vi "Measure.vi"() -> ()   [LabVIEW 2015]
uses:
  <vilib>/Utility/error.llb/DialogType.ctl
  <vilib>/DAQmx/write.llb/DAQmx Write (Analog 1D Wfm NChan NSamp).vi
  <vilib>/DAQmx/read.llb/DAQmx Read (Analog 1D Wfm NChan NSamp).vi
  <vilib>/DAQmx/create/channels.llb/DAQmx Create Channel (AO-Voltage-Basic).vi
  <vilib>/DAQmx/configure/timing.llb/DAQmx Timing (Sample Clock).vi
  <vilib>/DAQmx/create/channels.llb/DAQmx Create Channel (AI-Voltage-Basic).vi
  <vilib>/DAQmx/configure/trigger.llb/DAQmx Start Trigger (Digital Edge).vi
  <vilib>/DAQmx/miscellaneous.llb/DAQmx Fill In Error Info.vi
  <vilib>/measure/NI_MABase.lvlib
  <resource>/objmgr/daqmx.rc
panel:
  out "Waveform Chart":waveform(dbl)[](graph)
  in  "Samples to Read":i32=1000
  in  "rate":dbl=5000.0 caption="Update Generation Rate" format="%0.2f"
  in  "minimum value":dbl=-10.0 caption="Output Minimum Value" format="%0.2f"
  in  "maximum value":dbl=10.0 caption="Output Maximum Value" format="%0.2f"
  in  "Maximum Value":dbl=10.0 caption="Input Maximum Value" format="%0.2f"
  in  "Minimum Value":dbl=-10.0 caption="Input Minimum Value" format="%0.2f"
  in  "Rate":dbl=10000.0 caption="Input Rate" format="%0.2f"
  in  "?":bool
  in  "Fil lagres til":path
  in  "Ventetid(s)":u32
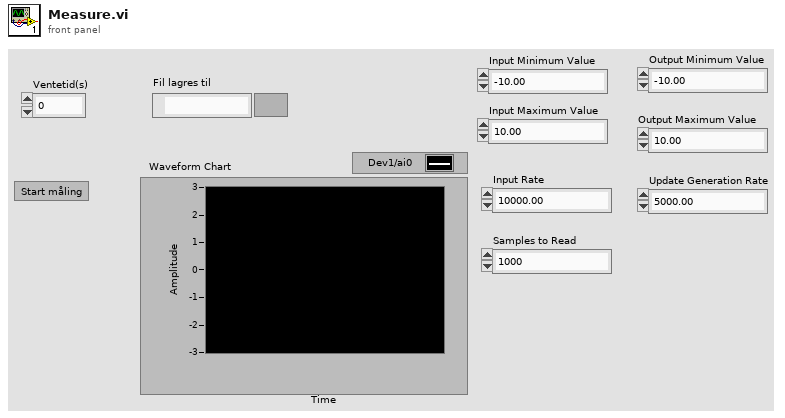
[diagram p1: front panel]
types:
  T1 = typedef "DialogType.ctl" = u16
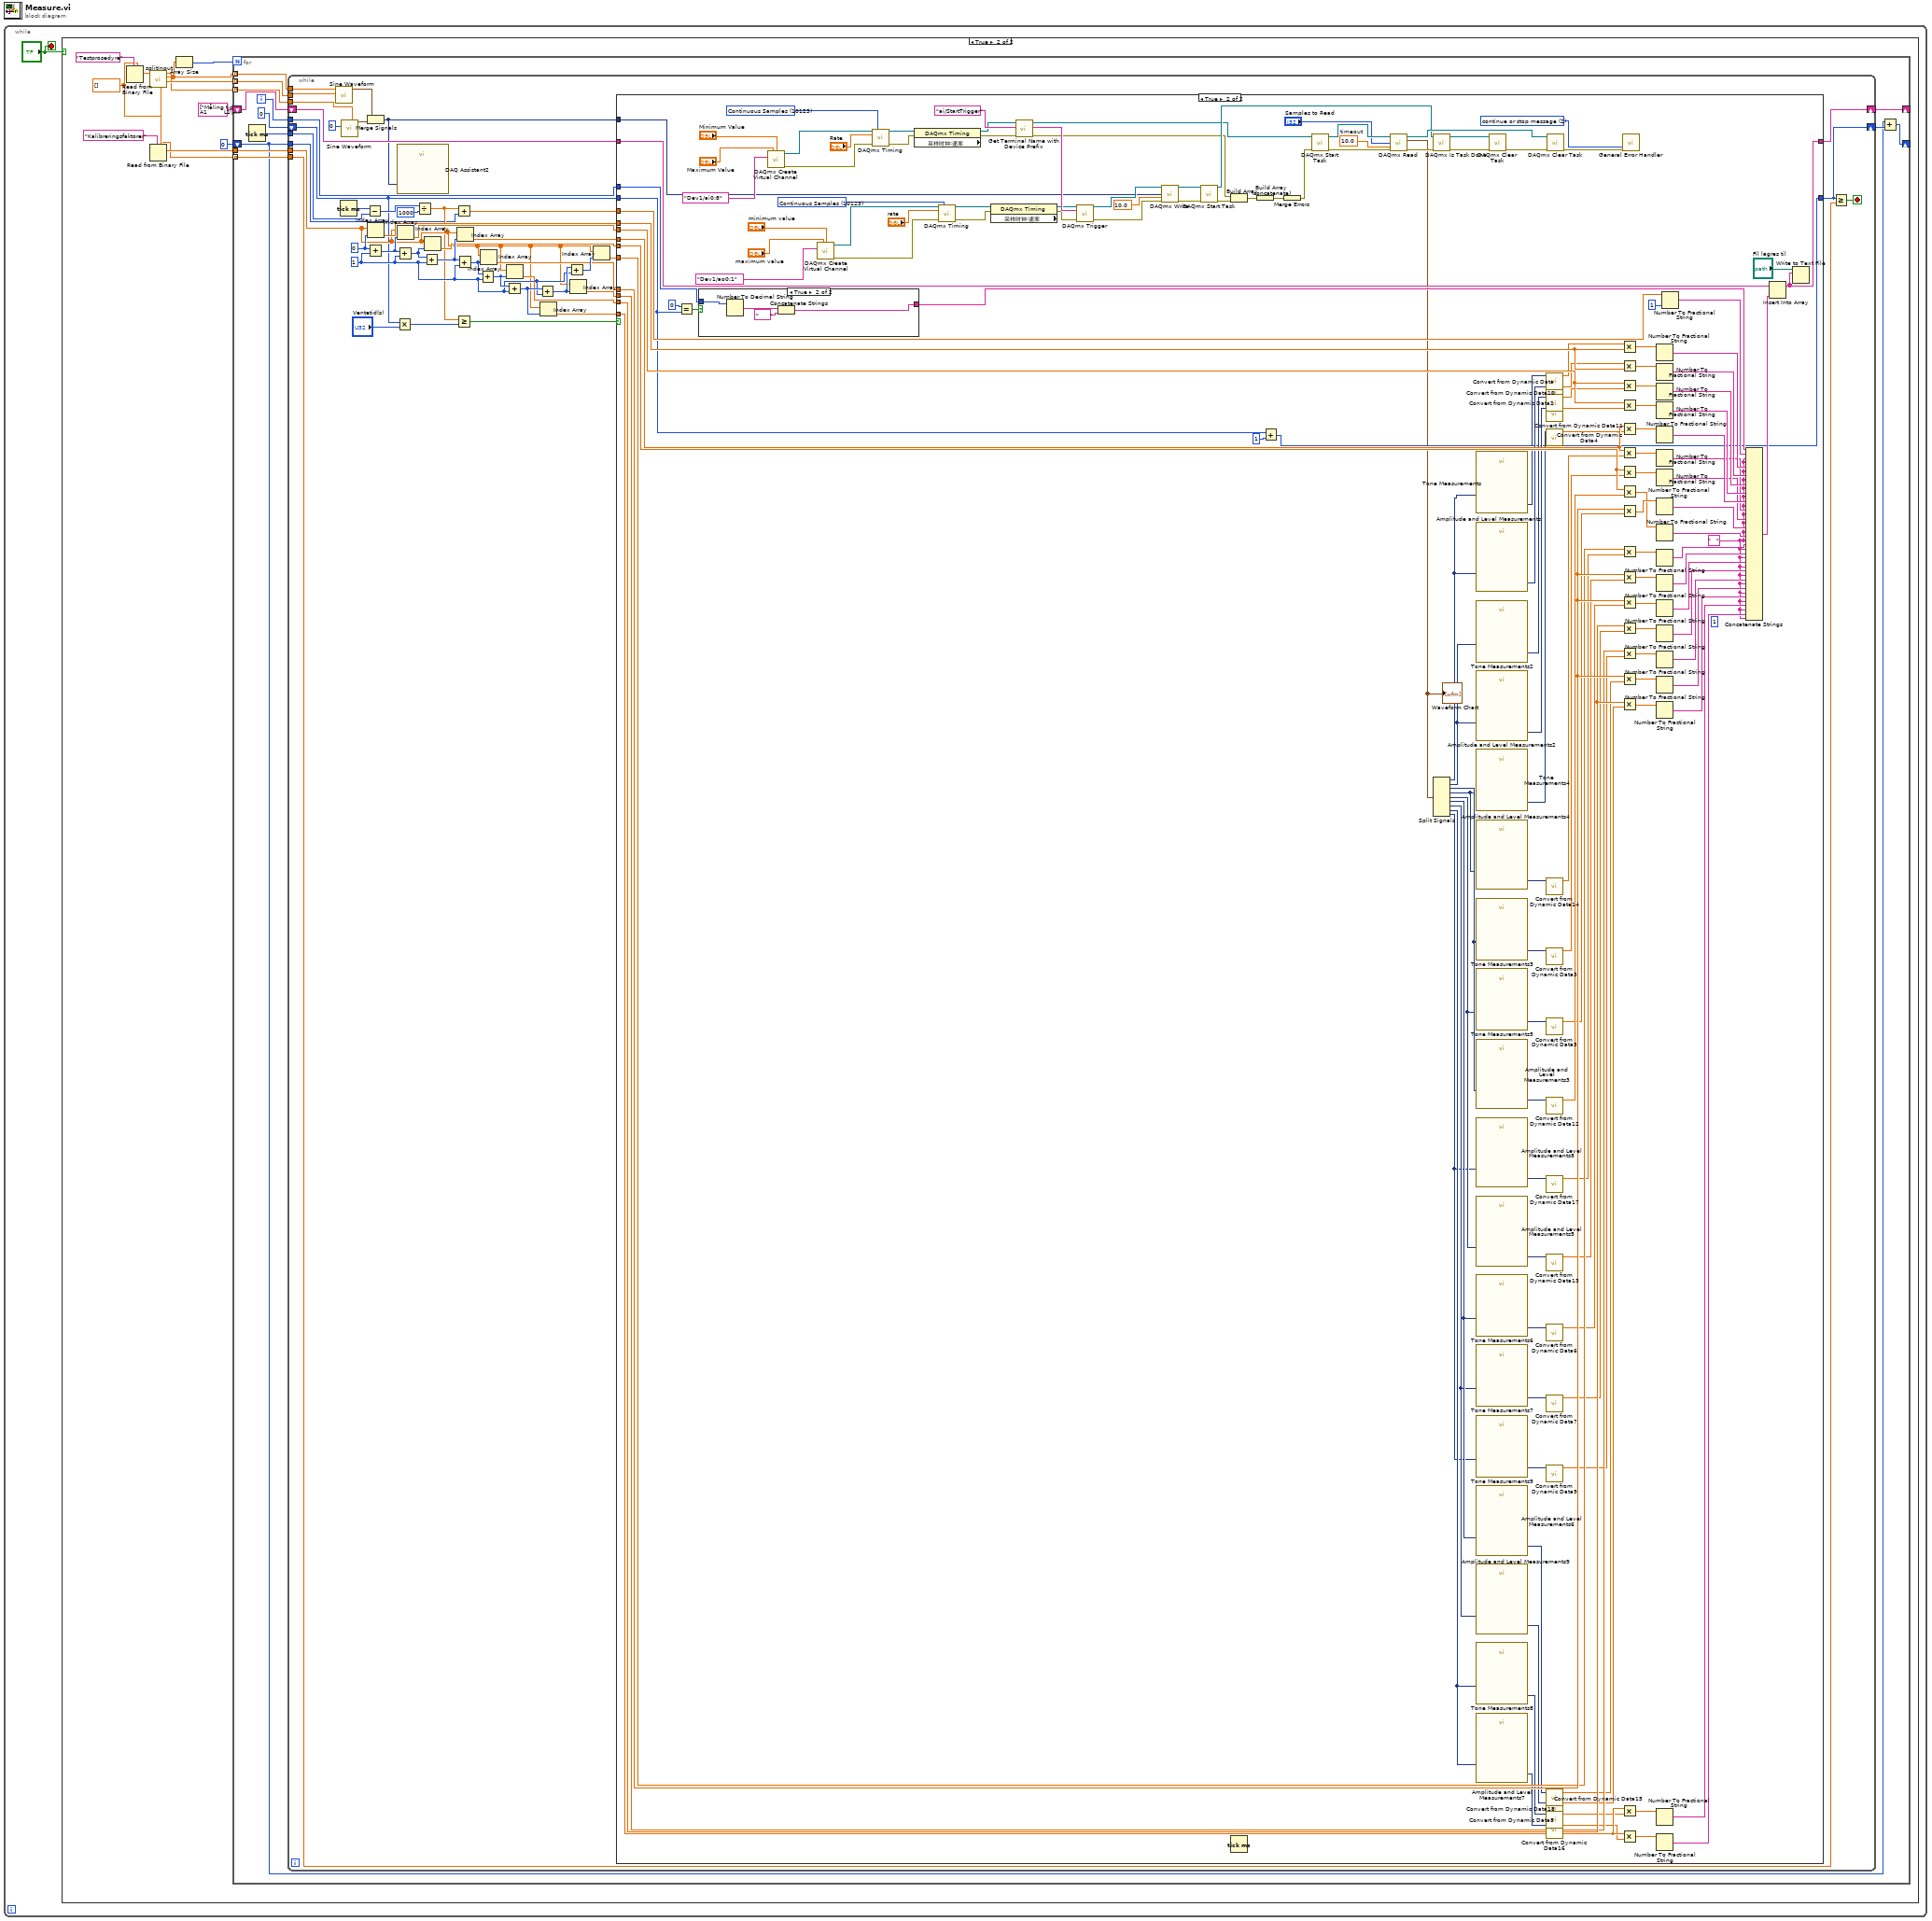
[diagram p0: block diagram]
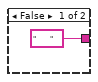
[diagram p4: hidden frame]
diagram:
  n1 = while {
    stop <- "?" stop-if-true
    n2 = case shown="True" "?" {
      frame False {
      }
      frame True {
        w9 = dbl[] [] ("Array")
        n3 = Read from Binary File(5:w9, 7:"Testprosedyre" ("String")) -> (2:w13:dbl[])  [unwired: 4 in, 3 out]
        n4 = call "splitInput.vi"("Array in"=w13) -> ("Amplitude"=w6:dbl[], "Frekvens"=w4:dbl[], "Temperatur"=w5:dbl[], "Perioder"=w7:dbl[])  [unwired: 7 in]
        n5 = Read from Binary File(5:w9, 7:"Kalibreringsfaktorer") -> (2:w8:dbl[])  [unwired: 4 in, 3 out]
        n6 = Array Size(array=w4) -> (size(s)=w11:i32)
        n7 = for {
          N: w11 -> [_]
          tunnel: w8 -> [w24]
          tunnel: w7 -> [w23] mode=indexing
          tunnel: w6 -> [w22] mode=indexing
          tunnel: w4 -> [w21] mode=indexing
          tunnel: w5 -> [w20] mode=indexing
          shift-right: [w18] -> _
          shift-left: string[] ["Måling tid       A1         L1\t       A2         L2         A3         L3         A4         L4         A5         L5         A6         L6         A7         L7         A8         L8         A9         L9"] ("Array") -> [w19]
          shift-right: [w14] -> _
          shift-left: 0 -> [w15]
          i -> [w25]
          n8 = Tick Count (ms)() -> (millisecond timer value=w17:u32)
          n9 = while {
            shift-right: [w42] -> w16
            shift-left: 0 -> [w36]
            shift-right: [w46] -> w18
            shift-left: w19 -> [w47]
            tunnel: w25 -> [w45]
            tunnel: w23 -> [w43]
            tunnel: w24 -> [w41]
            tunnel: w17 -> [w40]
            tunnel: w22 -> [w29]
            tunnel: w21 -> [w30]
            tunnel: w20 -> [w39]
            tunnel: w15 -> [w33]
            stop <- w44 stop-if-true
            w53 = 1
            w70 = 0
            n10 = call <vilib>:"Sine Waveform.vi"("amplitude"=w29, "frequency"=w30) -> ("signal out"=w27:waveform(dbl))  [unwired: 8 in, 1 out]
            n11 = Tick Count (ms)() -> (millisecond timer value=w50:u32)
            n12 = call <vilib>:"Sine Waveform.vi"("offset"=w39, "amplitude"=0) -> ("signal out"=w31:waveform(dbl))  [unwired: 8 in, 1 out]
            n13 = Subtract(x=w50, y=w40) -> (x-y=w49:u32)
            n14 = Add(x=w70, y=w53) -> (x+y=w52:i32)
            n15 = Merge Signals(w27, w31) -> (w32:dynamicdata)
            n16 = Index Array(array=w41, index=w70) -> (element=w62:dbl)
            n17 = Multiply(x=w36, y="Ventetid(s)") -> (x*y=w38:u32)
            n18 = Add(x=w52, y=w53) -> (x+y=w69:i32)
            n19 = call "DAQ Assistant2"("data"=w32) -> ()  [unwired: 17 in, 2 out]
            n20 = Index Array(array=w41, index=w52) -> (element=w61:dbl)
            n21 = Divide(x=w49, y=1000) -> (x/y=w34:dbl)
            n22 = Add(x=w69, y=w53) -> (x+y=w68:i32)
            n23 = Index Array(array=w41, index=w69) -> (element=w60:dbl)
            n24 = Add(x=w34, y=w33) -> (x+y=w35:dbl)
            n25 = Greater Or Equal?(x=w34, y=w38) -> (x >= y?=w48:bool)
            n26 = Add(x=w68, y=w53) -> (x+y=w67:i32)
            n27 = Index Array(array=w41, index=w68) -> (element=w59:dbl)
            n28 = Add(x=w67, y=w53) -> (x+y=w66:i32)
            n29 = Index Array(array=w41, index=w67) -> (element=w58:dbl)
            n30 = Add(x=w66, y=w53) -> (x+y=w65:i32)
            n31 = Index Array(array=w41, index=w66) -> (element=w57:dbl)
            n32 = Add(x=w65, y=w53) -> (x+y=w64:i32)
            n33 = Index Array(array=w41, index=w65) -> (element=w56:dbl)
            n34 = Add(x=w64, y=w53) -> (x+y=w63:i32)
            n35 = Index Array(array=w41, index=w64) -> (element=w55:dbl)
            n36 = Index Array(array=w41, index=w63) -> (element=w54:dbl)
            n37 = case shown="True" w48 {
              tunnel: w47 -> [w72 w226]
              tunnel: w62 -> [_ w225]
              tunnel: w61 -> [_ w224]
              tunnel: w60 -> [_ w223]
              tunnel: w59 -> [_ w222]
              tunnel: w58 -> [_ w221]
              tunnel: w57 -> [_ w220]
              tunnel: w56 -> [_ w219]
              tunnel: w55 -> [_ w218]
              tunnel: w54 -> [_ w217]
              tunnel: w35 -> [_ w129]
              tunnel: w36 -> [w71 w125]
              tunnel: [w72 w128] -> w46
              tunnel: w45 -> [_ w126]
              tunnel: [w71 w124] -> w42
              tunnel: w32 -> [_ w76]
              frame False {
              }
              frame True {
                (unwired) 1
                w79 = 10.0  # timeout
                w102 = T1 2 items=["no dialog", "OK message", "continue or stop message", "OK message + warnings", "continue/stop + warnings"] ("type of dialog (OK msg:1)")
                w114 = 10123 items=["Finite Samples"=10178, "Continuous Samples"=10123] ("sample mode")
                w120 = 10123 items=["Finite Samples"=10178, "Continuous Samples"=10123] ("sample mode")
                w130 = "   "
                n38 = Equal?(x=0, y=w125) -> (x = y?=w171:bool)
                n39 = case shown="True" w171 {
                  tunnel: ["       " w229] -> w151
                  tunnel: w126 -> [_ w228]
                  frame False {
                  }
                  frame True {
                    n40 = Number To Decimal String(number=w228) -> (decimal integer string=w231:string)  [unwired: 1 in]
                    n41 = Concatenate Strings(w231, "      ") -> (w229:string)
                  }
                }
                n42 = call-poly <vilib>:"DAQmx Create Virtual Channel.vi"("maximum value"="Maximum Value", "minimum value"="Minimum Value", "physical channels"=tag "Dev1/ai0:8" ("Physical Channel")) -> ("task out"=w118:refnum<k21>, "error out"=w119:errorcluster)  [unwired: 11 in]
                n43 = call-poly <vilib>:"DAQmx Create Virtual Channel.vi"("maximum value"="maximum value", "minimum value"="minimum value", "physical channels"=tag "Dev1/ao0:1") -> ("task out"=w113:refnum<k21>, "error out"=w112:errorcluster)  [unwired: 11 in]
                n44 = call-poly <vilib>:"DAQmx Timing.vi"("task/channels in"=w118, "sample mode"=w120, "rate"="Rate", "error in"=w119) -> ("task out"=w88:refnum<k21>, "error out"=w87:errorcluster)  [unwired: 10 in]
                n45 = property class="DAQmx Timing" props=["采样时钟:速率"](reference=w88, error in=w87) -> (reference out=w86:refnum<k21>, error out=w85:errorcluster)  [unwired: 1 out]
                n46 = call-poly <vilib>:"DAQmx Timing.vi"("task/channels in"=w113, "sample mode"=w114, "rate"="rate", "error in"=w112) -> ("task out"=w97:refnum<k21>, "error out"=w96:errorcluster)  [unwired: 10 in]
                n47 = property class="DAQmx Timing" props=["采样时钟:速率"](reference=w97, error in=w96) -> (reference out=w98:refnum<k21>, error out=w95:errorcluster)  [unwired: 1 out]
                n48 = call "Get Terminal Name with Device Prefix.vi"("error in (no error)"=w85, "Local Terminal Name"="ai/StartTrigger" ("terminal"), "task/channels in"=w86) -> ("error out"=w92:errorcluster, "Terminal Name with Device Prefix"=w99:tag, "task out"=w94:refnum<k21>)  [unwired: 6 in]
                n49 = call-poly <vilib>:"DAQmx Trigger.vi"("task/channels in"=w98, "source"=w99, "error in"=w95) -> ("task out"=w104:refnum<k21>, "error out"=w105:errorcluster)  [unwired: 11 in]
                n50 = call-poly <vilib>:"DAQmx Write.vi"("task/channels in"=w104, "data"=w76, "timeout"=10.0 ("Wirite Timeout"), "error in"=w105) -> ("task out"=w107:refnum<k21>, "error out"=w106:errorcluster)  [unwired: 9 in, 1 out]
                n51 = call <vilib>:"DAQmx Start Task.vi"("task/channels in"=w107, "error in"=w106) -> ("task out"=w111:refnum<k21>, "error out"=w91:errorcluster)  [unwired: 12 in]
                n52 = Build Array(w92, w91) -> (w81:errorcluster[])
                n53 = Tick Count (ms)() -> ()  [unwired: 1 out]
                n54 = Build Array (concatenate)(w81) -> (w80:errorcluster[])
                n55 = Add(x=w125, y=1) -> (x+y=w124:i32)
                n56 = Merge Errors(w80) -> (w90:errorcluster)
                n57 = call <vilib>:"DAQmx Start Task.vi"("task/channels in"=w94, "error in"=w90) -> ("task out"=w93:refnum<k21>, "error out"=w89:errorcluster)  [unwired: 12 in]
                n58 = call-poly <vilib>:"DAQmx Read.vi"("task/channels in"=w93, "number of samples per channel"="Samples to Read", "timeout"=w79, "error in"=w89) -> ("task out"=w121:refnum<k21>, "data"=w73:waveform(dbl)[], "error out"=w77:errorcluster)  [unwired: 9 in]
                "Waveform Chart" <- w73
                n59 = call <vilib>:"DAQmx Is Task Done.vi"("task/channels in"=w111, "error in"=w77) -> ("task out"=w110:refnum<k21>, "error out"=w84:errorcluster)  [unwired: 11 in, 1 out]
                n60 = Split Signals(w73) -> (w74:dynamicdata, w180:dynamicdata, w179:dynamicdata, w178:dynamicdata, w177:dynamicdata, w176:dynamicdata, w175:dynamicdata, w174:dynamicdata, w173:dynamicdata)  [unwired: 9 in]
                n61 = call "Tone Measurements"("Signals"=w74) -> ("Amplitude"=w75:dynamicdata)  [unwired: 9 in, 1 out]
                n62 = call "Amplitude and Level Measurements"("Signals"=w74) -> ("Mean (DC)"=w189:dynamicdata)  [unwired: 13 in, 1 out]
                n63 = call "Tone Measurements2"("Signals"=w180) -> ("Amplitude"=w197:dynamicdata)  [unwired: 9 in, 1 out]
                n64 = call "Amplitude and Level Measurements2"("Signals"=w180) -> ("Mean (DC)"=w188:dynamicdata)  [unwired: 13 in, 1 out]
                n65 = call "Tone Measurements4"("Signals"=w178) -> ("Amplitude"=w195:dynamicdata)  [unwired: 9 in, 1 out]
                n66 = call "Amplitude and Level Measurements4"("Signals"=w178) -> ("Mean (DC)"=w185:dynamicdata)  [unwired: 13 in, 1 out]
                n67 = call "Tone Measurements3"("Signals"=w179) -> ("Amplitude"=w196:dynamicdata)  [unwired: 9 in, 1 out]
                n68 = call "Tone Measurements5"("Signals"=w177) -> ("Amplitude"=w194:dynamicdata)  [unwired: 9 in, 1 out]
                n69 = call "Amplitude and Level Measurements3"("Signals"=w179) -> ("Mean (DC)"=w187:dynamicdata)  [unwired: 13 in, 1 out]
                n70 = call "Amplitude and Level Measurements8"("Signals"=w173) -> ("Mean (DC)"=w182:dynamicdata)  [unwired: 13 in, 1 out]
                n71 = call "Amplitude and Level Measurements5"("Signals"=w177) -> ("Mean (DC)"=w186:dynamicdata)  [unwired: 13 in, 1 out]
                n72 = call "Tone Measurements6"("Signals"=w176) -> ("Amplitude"=w193:dynamicdata)  [unwired: 9 in, 1 out]
                n73 = call "Tone Measurements7"("Signals"=w175) -> ("Amplitude"=w192:dynamicdata)  [unwired: 9 in, 1 out]
                n74 = call "Tone Measurements9"("Signals"=w173) -> ("Amplitude"=w190:dynamicdata)  [unwired: 9 in, 1 out]
                n75 = call "Amplitude and Level Measurements6"("Signals"=w176) -> ("Mean (DC)"=w184:dynamicdata)  [unwired: 13 in, 1 out]
                n76 = call "Amplitude and Level Measurements9"("Signals"=w175) -> ("Mean (DC)"=w181:dynamicdata)  [unwired: 13 in, 1 out]
                n77 = call "Tone Measurements8"("Signals"=w174) -> ("Amplitude"=w191:dynamicdata)  [unwired: 9 in, 1 out]
                n78 = call "Amplitude and Level Measurements7"("Signals"=w174) -> ("Mean (DC)"=w183:dynamicdata)  [unwired: 13 in, 1 out]
                n79 = call <vilib>:"DAQmx Clear Task.vi"("task in"=w110, "error in"=w84) -> ("error out"=w83:errorcluster)  [unwired: 13 in]
                n80 = call "Convert from Dynamic Data"("Dynamic Data Type"=w75) -> ("Scalar"=w215:dbl)  [unwired: 3 in]
                n81 = call "Convert from Dynamic Data10"("Dynamic Data Type"=w189) -> ("Scalar"=w213:dbl)  [unwired: 3 in]
                n82 = call "Convert from Dynamic Data2"("Dynamic Data Type"=w197) -> ("Scalar"=w214:dbl)  [unwired: 3 in]
                n83 = call "Convert from Dynamic Data11"("Dynamic Data Type"=w188) -> ("Scalar"=w212:dbl)  [unwired: 3 in]
                n84 = call "Convert from Dynamic Data4"("Dynamic Data Type"=w195) -> ("Scalar"=w209:dbl)  [unwired: 3 in]
                n85 = call "Convert from Dynamic Data14"("Dynamic Data Type"=w185) -> ("Scalar"=w208:dbl)  [unwired: 3 in]
                n86 = call "Convert from Dynamic Data3"("Dynamic Data Type"=w196) -> ("Scalar"=w211:dbl)  [unwired: 3 in]
                n87 = call "Convert from Dynamic Data5"("Dynamic Data Type"=w194) -> ("Scalar"=w207:dbl)  [unwired: 3 in]
                n88 = call "Convert from Dynamic Data12"("Dynamic Data Type"=w187) -> ("Scalar"=w210:dbl)  [unwired: 3 in]
                n89 = call "Convert from Dynamic Data17"("Dynamic Data Type"=w182) -> ("Scalar"=w198:dbl)  [unwired: 3 in]
                n90 = call "Convert from Dynamic Data13"("Dynamic Data Type"=w186) -> ("Scalar"=w206:dbl)  [unwired: 3 in]
                n91 = call "Convert from Dynamic Data6"("Dynamic Data Type"=w193) -> ("Scalar"=w205:dbl)  [unwired: 3 in]
                n92 = call "Convert from Dynamic Data7"("Dynamic Data Type"=w192) -> ("Scalar"=w202:dbl)  [unwired: 3 in]
                n93 = call "Convert from Dynamic Data9"("Dynamic Data Type"=w190) -> ("Scalar"=w199:dbl)  [unwired: 3 in]
                n94 = call "Convert from Dynamic Data15"("Dynamic Data Type"=w184) -> ("Scalar"=w204:dbl)  [unwired: 3 in]
                n95 = call "Convert from Dynamic Data18"("Dynamic Data Type"=w181) -> ("Scalar"=w203:dbl)  [unwired: 3 in]
                n96 = call "Convert from Dynamic Data8"("Dynamic Data Type"=w191) -> ("Scalar"=w200:dbl)  [unwired: 3 in]
                n97 = call "Convert from Dynamic Data16"("Dynamic Data Type"=w183) -> ("Scalar"=w201:dbl)  [unwired: 3 in]
                n98 = call <vilib>:"DAQmx Clear Task.vi"("task in"=w121, "error in"=w83) -> ("error out"=w82:errorcluster)  [unwired: 13 in]
                n99 = Multiply(x=w215, y=w225) -> (x*y=w169:dbl)
                n100 = Multiply(x=w213, y=w225) -> (x*y=w168:dbl)
                n101 = Multiply(x=w224, y=w214) -> (x*y=w167:dbl)
                n102 = Multiply(x=w224, y=w212) -> (x*y=w166:dbl)
                n103 = Multiply(x=w222, y=w209) -> (x*y=w165:dbl)
                n104 = Multiply(x=w222, y=w208) -> (x*y=w164:dbl)
                n105 = Multiply(x=w223, y=w211) -> (x*y=w163:dbl)
                n106 = Multiply(x=w223, y=w210) -> (x*y=w161:dbl)
                n107 = Multiply(x=w221, y=w207) -> (x*y=w162:dbl)
                n108 = Multiply(x=w217, y=w198) -> (x*y=w152:dbl)
                n109 = Multiply(x=w221, y=w206) -> (x*y=w153:dbl)
                n110 = Multiply(x=w221, y=w205) -> (x*y=w154:dbl)
                n111 = Multiply(x=w220, y=w202) -> (x*y=w155:dbl)
                n112 = Multiply(x=w218, y=w199) -> (x*y=w156:dbl)
                n113 = Multiply(x=w221, y=w204) -> (x*y=w157:dbl)
                n114 = Multiply(x=w220, y=w203) -> (x*y=w158:dbl)
                n115 = Multiply(x=w219, y=w200) -> (x*y=w159:dbl)
                n116 = Multiply(x=w219, y=w201) -> (x*y=w160:dbl)
                n117 = call <vilib>:"General Error Handler.vi"("type of dialog (OK msg:1)"=w102, "error in (no error)"=w82) -> ()  [unwired: 9 in, 5 out]
                n118 = Number To Fractional String(number=w169) -> (F-format string=w150:string)  [unwired: 3 in]
                n119 = Number To Fractional String(number=w168) -> (F-format string=w149:string)  [unwired: 3 in]
                n120 = Number To Fractional String(number=w167) -> (F-format string=w148:string)  [unwired: 3 in]
                n121 = Number To Fractional String(number=w166) -> (F-format string=w147:string)  [unwired: 3 in]
                n122 = Number To Fractional String(number=w165) -> (F-format string=w146:string)  [unwired: 3 in]
                n123 = Number To Fractional String(number=w164) -> (F-format string=w145:string)  [unwired: 3 in]
                n124 = Number To Fractional String(number=w163) -> (F-format string=w144:string)  [unwired: 3 in]
                n125 = Number To Fractional String(number=w162) -> (F-format string=w143:string)  [unwired: 3 in]
                n126 = Number To Fractional String(number=w161) -> (F-format string=w142:string)  [unwired: 3 in]
                n127 = Number To Fractional String(number=w152) -> (F-format string=w141:string)  [unwired: 3 in]
                n128 = Number To Fractional String(number=w153) -> (F-format string=w140:string)  [unwired: 3 in]
                n129 = Number To Fractional String(number=w154) -> (F-format string=w139:string)  [unwired: 3 in]
                n130 = Number To Fractional String(number=w155) -> (F-format string=w138:string)  [unwired: 3 in]
                n131 = Number To Fractional String(number=w156) -> (F-format string=w137:string)  [unwired: 3 in]
                n132 = Number To Fractional String(number=w157) -> (F-format string=w136:string)  [unwired: 3 in]
                n133 = Number To Fractional String(number=w158) -> (F-format string=w135:string)  [unwired: 3 in]
                n134 = Number To Fractional String(number=w159) -> (F-format string=w134:string)  [unwired: 3 in]
                n135 = Number To Fractional String(number=w160) -> (F-format string=w133:string)  [unwired: 3 in]
                n136 = Number To Fractional String(number=w129, precision (6)=1) -> (F-format string=w131:string)  [unwired: 2 in]
                n137 = Concatenate Strings(w151, w131, w130, w130, w150, w130, w149, w130, w148, w130, w147, w130, w146, w130, w145, w130, w144, w130, w143, w130, w142, w130, w141, w130, w140, w130, w139, w130, w138, w130, w137, w130, w136, w130, w135, w130, w134, w130, w133, w130) -> (w132:string)
                n138 = Insert Into Array(array=w226, new element=w132) -> (w128:string[])  [unwired: 1 in]
                n139 = Write to Text File(file (use dialog)="Fil lagres til", text=w128) -> ()  [unwired: 2 in, 3 out]
              }
            }
            n140 = Greater Or Equal?(x=w42, y=w43) -> (x >= y?=w44:bool)
          }
          n141 = Add(x=w15, y=w16) -> (x+y=w14:i32)
        }
      }
    }
  }
